vi "Add LVCLASS-Tag.vi"(1 "LVClass Name":string) -> (0 "Tagged LVClass Name":string)   [LabVIEW 2014, in "CS++Utilities.lvlib"]
doc: "Surround LV classname with Tags <LVCLASS>classname</LVCLASS>."
uses:
  CS++Utilities.lvlib
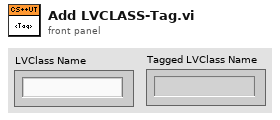
[diagram p1: front panel]
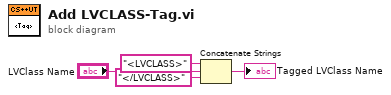
[diagram p0: block diagram]
diagram:
  n1 = Concatenate Strings("<LVCLASS>" ("string"), "LVClass Name", "</LVCLASS>" ("string")) -> (→"Tagged LVClass Name":string)
